vi "UI Initialize.vi"(8 "error in (no error)":errorcluster, 11 "New Project Wizard in":refnum<class "Update Project Wizard.lvclass">) -> (0 "error out":errorcluster, 3 "New Project Wizard out":refnum<class "Update Project Wizard.lvclass">)   [LabVIEW 2013, in "SET Project Editor.lvlib" / "Update Project Wizard.lvclass"]
uses:
  Update Project Wizard.lvclass
  Update Project Wizard.lvclass/Update Project Wizard.ctl
  UI Wizard/UI Wizard.lvclass
  SET Project Editor.lvlib
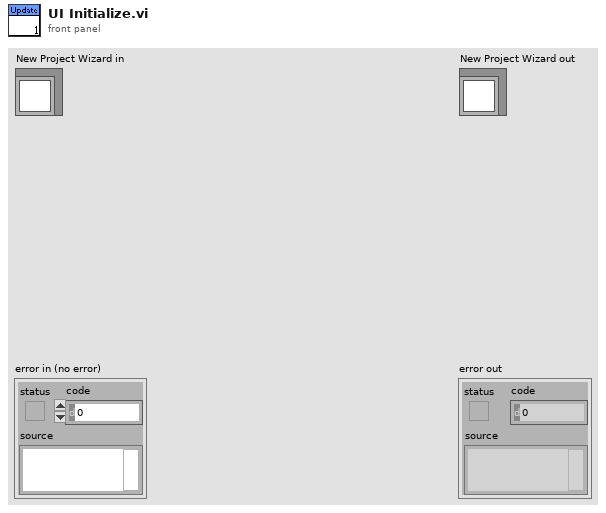
[diagram p1: front panel]
types:
  T1 = enum32{"Invalid", "Default", "Floating", "Floating/Auto-Hide", "Modal"}
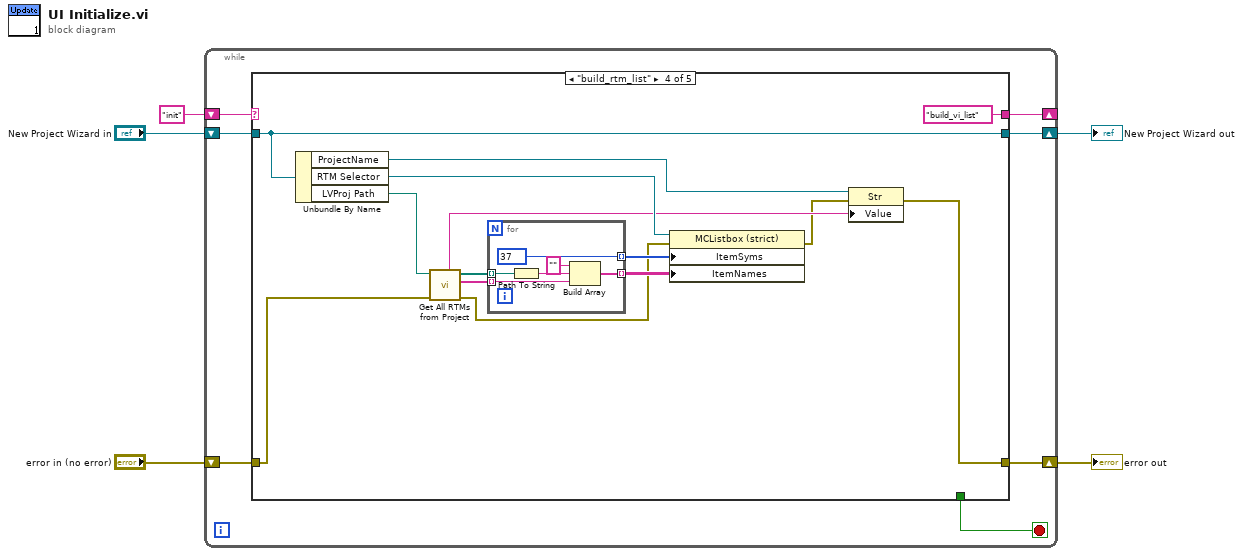
[diagram p0: block diagram]
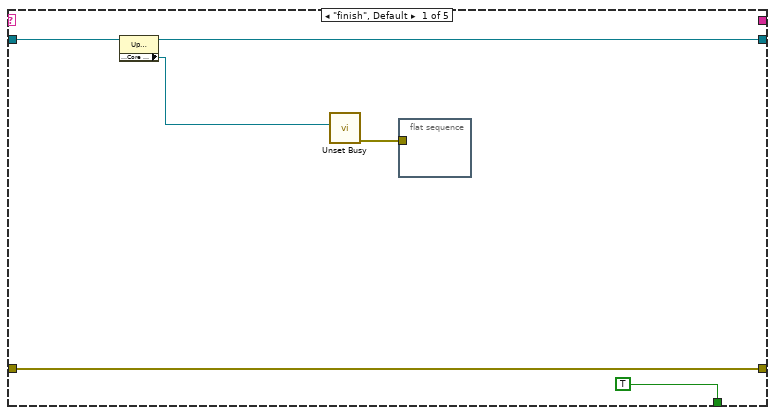
[diagram p2: hidden frame]
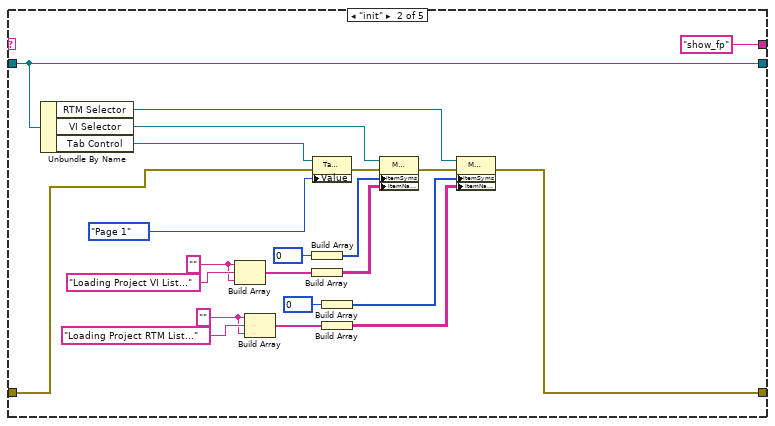
[diagram p3: hidden frame]
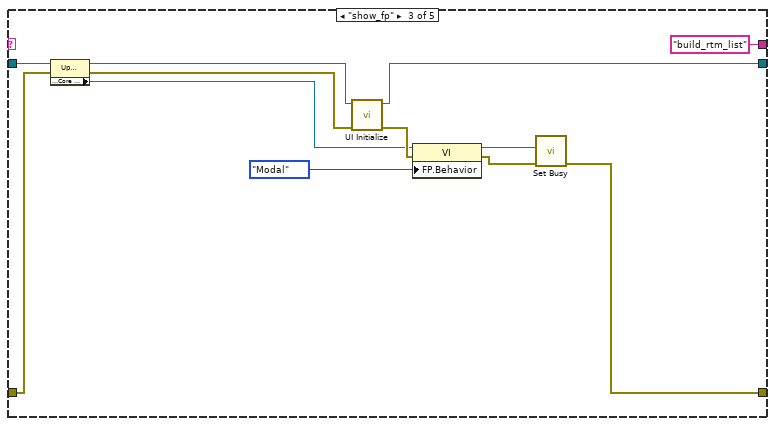
[diagram p4: hidden frame]
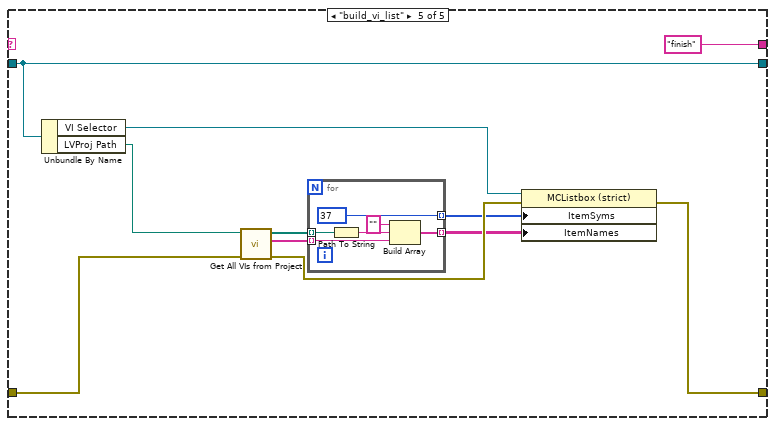
[diagram p5: hidden frame]
diagram:
  n1 = while {
    shift-right: [w8] -> w1
    shift-left: "New Project Wizard in" -> [w12]
    shift-right: [w7] -> _
    shift-left: "init" -> [w11]
    shift-right: [w9] -> w2
    shift-left: "error in (no error)" -> [w10]
    stop <- w6 stop-if-true
    n2 = case shown="\"build_rtm_list\"" w11 {
      tunnel: w12 -> [w16 w21 w50 w56 w74]
      tunnel: w10 -> [w18 w19 w47 w61 w75]
      tunnel: [w18 w22 w42 w54 w78] -> w9
      tunnel: [w15 w21 w45 w56 w74] -> w8
      tunnel: [_ "show_fp" "build_rtm_list" "build_vi_list" "finish"] -> w7
      tunnel: [TRUE _ _ _ _] -> w6
      frame "finish", Default {
        n3 = property class="Update Project Wizard.lvclass"(reference=w16) -> (reference out=w15:refnum<class "Update Project Wizard.lvclass">, "Properties:Core VI Refnum"=w14:refnum<vi>)  [unwired: 1 in, 1 out]
        n4 = call <vilib>:"Unset Busy.vi"("VI reference (current VI)"=w14) -> ("error out"=w17:errorcluster)  [unwired: 10 in]
        n5 = flat-sequence {
          tunnel: w17 -> [_]
          frame #0 {
          }
        }
      }
      frame "init" {
        w29 = ""
        w35 = ""
        n6 = Unbundle By Name(w21) -> ("RTM Selector"=w26:refnum<vi>, "VI Selector"=w34:refnum<vi>, "Tab Control"=w39:refnum<vi>)
        n7 = Build Array(w35, "Loading Project VI List...", w35) -> (w38:string[])
        n8 = Build Array(w29, "Loading Project RTM List...", w29) -> (w31:string[])
        n9 = Build Array(0) -> (w28:i32[])
        n10 = Build Array(w38) -> (w27:string[][])
        n11 = property class="TabCtl (strict)"(reference=w39, error in=w19, "Value"=enum32{"Page 1", "Page 2"}."Page 1") -> (error out=w33:errorcluster)  [unwired: 1 out]
        n12 = Build Array(0) -> (w25:i32[])
        n13 = Build Array(w31) -> (w24:string[][])
        n14 = property on="Property Node" class="MCListbox (strict)"(reference=w34, error in=w33, "ItemSyms"=w28, "ItemNames"=w27) -> (error out=w23:errorcluster)  [unwired: 1 out]
        n15 = property on="Property Node" class="MCListbox (strict)"(reference=w26, error in=w23, "ItemSyms"=w25, "ItemNames"=w24) -> (error out=w22:errorcluster)  [unwired: 1 out]
      }
      frame "show_fp" {
        n16 = property class="Update Project Wizard.lvclass"(reference=w50, error in=w47) -> (reference out=w48:refnum<class "Update Project Wizard.lvclass">, error out=w46:errorcluster, "Properties:Core VI Refnum"=w49:refnum<vi>)
        n17 = call-parent "UI Initialize.vi"("error in (no error)"=w46, "UI Wizard in"=w48) -> ("error out"=w51:errorcluster, "UI Wizard out"=w45:refnum<class "Update Project Wizard.lvclass">)  [unwired: 8 in]
        n18 = property class="VI"(reference=w49, error in=w51, "FP.Behavior"=T1."Modal" ("Front Panel Window:Behavior")) -> (reference out=w44:refnum<vi>, error out=w43:errorcluster)
        n19 = call <vilib>:"Set Busy.vi"("error in (no error)"=w43, "VI reference (current VI)"=w44) -> ("error out"=w42:errorcluster)  [unwired: 8 in, 1 out]
      }
      frame "build_rtm_list" {
        n20 = Unbundle By Name(w56) -> ("ProjectName"=w60:refnum<vi>, "RTM Selector"=w59:refnum<vi>, "LVProj Path"=w62:path)
        n21 = call "Get All RTMs from Project.vi"("error in (no error)"=w61, "Project Path"=w62) -> ("error out"=w58:errorcluster, "RTM Virtual Paths"=w64:string[], "Project RTMs"=w63:path[], "Project Name"=w57:string)  [unwired: 6 in]
        n22 = for {
          tunnel: w63 -> [w72] mode=indexing
          tunnel: w64 -> [w70] mode=indexing
          tunnel: [w68] -> w66 mode=indexing
          tunnel: [37] -> w65 mode=indexing
          n23 = Path To String(path=w72) -> (string=w71:string)
          n24 = Build Array("" ("element"), w71, w70) -> (w68:string[])
        }
        n25 = property on="Property Node" class="MCListbox (strict)"(reference=w59, error in=w58, "ItemSyms"=w65, "ItemNames"=w66) -> (error out=w55:errorcluster)  [unwired: 1 out]
        n26 = property class="Str"(reference=w60, error in=w55, "Value"=w57) -> (error out=w54:errorcluster)  [unwired: 1 out]
      }
      frame "build_vi_list" {
        n27 = Unbundle By Name(w74) -> ("VI Selector"=w77:refnum<vi>, "LVProj Path"=w76:path)
        n28 = call "Get All VIs from Project.vi"("error in (no error)"=w75, "Project Path"=w76) -> ("error out"=w83:errorcluster, "VI Virtual Paths"=w79:string[], "Project VIs"=w80:path[])  [unwired: 6 in, 1 out]
        n29 = for {
          tunnel: w80 -> [w89] mode=indexing
          tunnel: w79 -> [w87] mode=indexing
          tunnel: [w85] -> w82 mode=indexing
          tunnel: [37] -> w81 mode=indexing
          n30 = Path To String(path=w89) -> (string=w88:string)
          n31 = Build Array("" ("element"), w88, w87) -> (w85:string[])
        }
        n32 = property on="Property Node" class="MCListbox (strict)"(reference=w77, error in=w83, "ItemSyms"=w81, "ItemNames"=w82) -> (error out=w78:errorcluster)  [unwired: 1 out]
      }
    }
  }
  "error out" <- w2
  "New Project Wizard out" <- w1
